vi "Motor Init.vi"(8 "Error in":errorcluster caption="错误输入（无错误）", 11 "VISA资源名称":refnum<visa-resource-name>) -> (0 "Error out":errorcluster caption="错误输出")   [LabVIEW 2017]
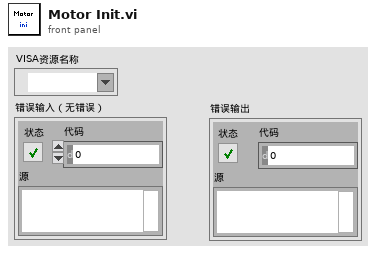
[diagram p1: front panel]
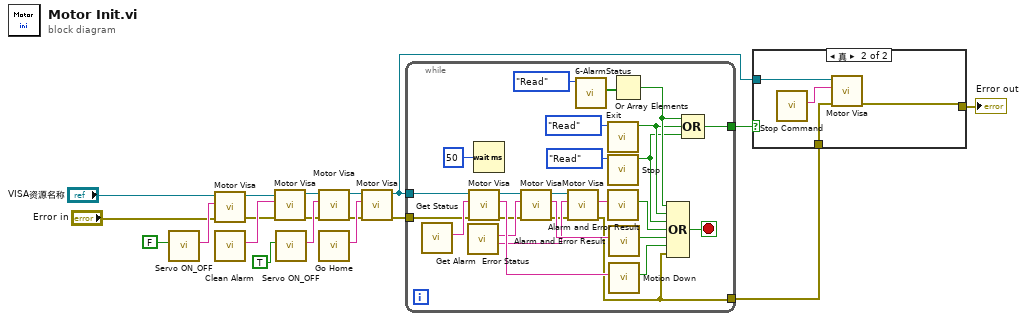
[diagram p0: block diagram]
diagram:
  n1 = call "Servo ON_OFF.vi"("Servo ON/OFF"=FALSE) -> ("Command"=w9:string)  [unwired: 10 in]
  n2 = call "Motor Visa.vi"("错误输入（无错误）"="Error in", "Command"=w9, "VISA资源名称"="VISA资源名称") -> ("错误输出"=w5:errorcluster, "VISA资源名称输出"=w10:refnum<visa-resource-name>)  [unwired: 6 in, 1 out]
  n3 = call "Clean Alarm.vi"() -> ("Clean Alarm"=w15:string)  [unwired: 11 in]
  n4 = call "Motor Visa.vi"("错误输入（无错误）"=w5, "Command"=w15, "VISA资源名称"=w10) -> ("错误输出"=w4:errorcluster, "VISA资源名称输出"=w14:refnum<visa-resource-name>)  [unwired: 6 in, 1 out]
  n5 = call "Servo ON_OFF.vi"("Servo ON/OFF"=TRUE) -> ("Command"=w19:string)  [unwired: 10 in]
  n6 = call "Motor Visa.vi"("错误输入（无错误）"=w4, "Command"=w19, "VISA资源名称"=w14) -> ("错误输出"=w3:errorcluster, "VISA资源名称输出"=w16:refnum<visa-resource-name>)  [unwired: 6 in, 1 out]
  n7 = call "Go Home.vi"() -> ("Go Home"=w17:string)  [unwired: 11 in]
  n8 = call "Motor Visa.vi"("错误输入（无错误）"=w3, "Command"=w17, "VISA资源名称"=w16) -> ("错误输出"=w2:errorcluster, "VISA资源名称输出"=w12:refnum<visa-resource-name>)  [unwired: 6 in, 1 out]
  n9 = while {
    tunnel: w12 -> [w44]
    tunnel: [w24] -> w13
    tunnel: w2 -> [w23]
    tunnel: [w20] -> w1
    stop <- w34 stop-if-true
    n10 = call "Get Status.vi"() -> ("Command"=w45:string)  [unwired: 11 in]
    n11 = call "Get Alarm  Error Status.vi"() -> ("AlarmStatus"=w37:string, "ErrorStatus"=w38:string)  [unwired: 10 in]
    n12 = call "Motor Visa.vi"("错误输入（无错误）"=w23, "Command"=w45, "VISA资源名称"=w44) -> ("错误输出"=w22:errorcluster, "读取缓冲区"=w43:string, "VISA资源名称输出"=w36:refnum<visa-resource-name>)  [unwired: 6 in]
    n13 = Wait (ms)(milliseconds to wait=u32 50 ("等待时间（毫秒）")) -> ()  [unwired: 1 out]
    n14 = call "Motor Visa.vi"("错误输入（无错误）"=w22, "Command"=w38, "VISA资源名称"=w36) -> ("错误输出"=w21:errorcluster, "读取缓冲区"=w40:string, "VISA资源名称输出"=w41:refnum<visa-resource-name>)  [unwired: 6 in]
    n15 = call "Motor Visa.vi"("错误输入（无错误）"=w21, "Command"=w37, "VISA资源名称"=w41) -> ("错误输出"=w20:errorcluster, "读取缓冲区"=w39:string)  [unwired: 6 in, 1 out]
    n16 = call "6-AlarmStatus.vi"("Step"=enum16{"Initial", "Write", "Read"}."Read") -> ("AlarmValue Out"=w28:bool[])  [unwired: 9 in, 1 out]
    n17 = call "Exit.vi"("Step"=enum16{"Initial", "Write", "Read"}."Read" ("step")) -> ("Exit Out"=w26:bool)  [unwired: 9 in, 1 out]
    n18 = call "Stop.vi"("Step"=enum16{"Initial", "Write", "Read"}."Read") -> ("Stop Out"=w25:bool)  [unwired: 9 in, 1 out]
    n19 = call "Alarm and Error Result.vi"("Command"=w39) -> ("Alarm or Error"=w31:bool)  [unwired: 10 in]
    n20 = call "Alarm and Error Result.vi"("Command"=w40) -> ("Alarm or Error"=w30:bool)  [unwired: 10 in]
    n21 = call "Motion Down.vi"("Command"=w43) -> ("Motion Down"=w35:bool)  [unwired: 10 in]
    n22 = Or Array Elements(Boolean array=w28) -> (logical OR=w27:bool)
    n23 = Compound Arithmetic op=OR(w27, w26, w25, w31, w30, w35, w20) -> (w34:bool)
    n24 = Compound Arithmetic op=OR(w27, w26, w25) -> (w24:bool)
  }
  n25 = case shown="真" w13 {
    tunnel: w12 -> [_ w49]
    tunnel: [w46 w48] -> w6
    tunnel: w1 -> [w46 w47]
    frame False {
    }
    frame True {
      n26 = call "Stop Command.vi"() -> ("Stop"=w50:string)  [unwired: 11 in]
      n27 = call "Motor Visa.vi"("错误输入（无错误）"=w47, "Command"=w50, "VISA资源名称"=w49) -> ("错误输出"=w48:errorcluster)  [unwired: 6 in, 2 out]
    }
  }
  "Error out" <- w6
